vi "Retrieve Buffered Currents.vi"(0 "VISA resource name in":refnum<visa-resource-name>, 7 "Expected Points?":i32, 11 "error in":errorcluster) -> (4 "VISA resource name out":refnum<visa-resource-name>, 8 "Current Data":sgl[](array[numeric]), 15 "error out":errorcluster)   [LabVIEW 2010]
uses:
  <instrlib>/Keithley 2400/Keithley 24XX.lvlib
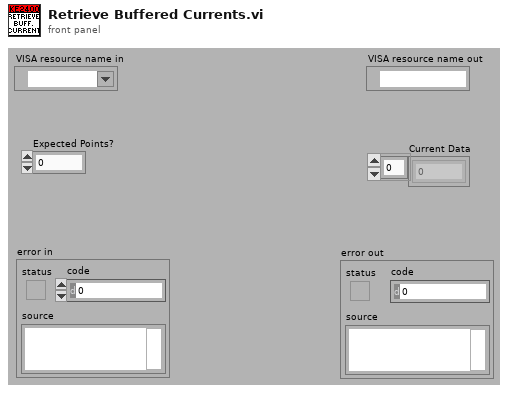
[diagram p1: front panel]
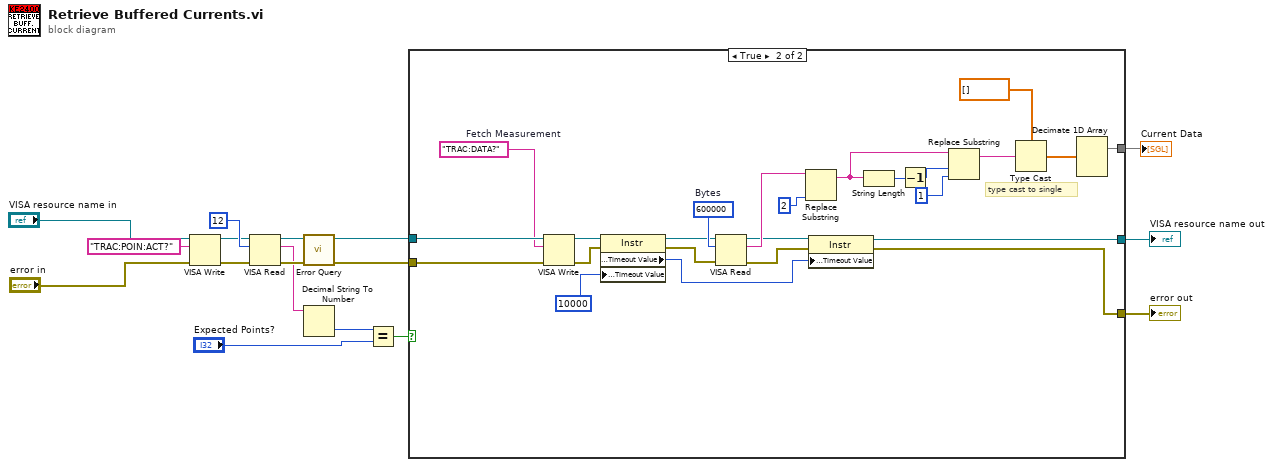
[diagram p0: block diagram]
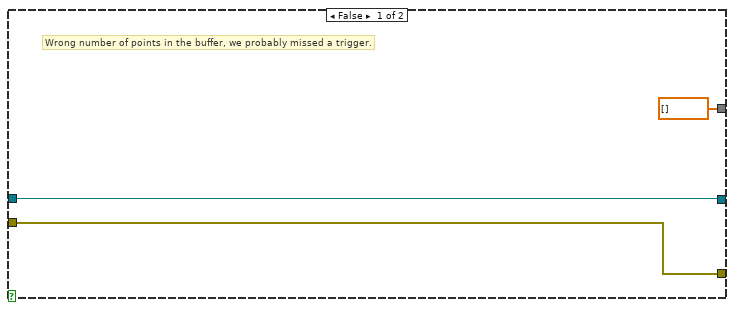
[diagram p2: hidden frame]
diagram:
  n1 = VISA Write(VISA resource name="VISA resource name in", write buffer="TRAC:POIN:ACT?", error in (no error)="error in") -> (VISA resource name out=w9:refnum<visa-resource-name>, error out=w8:errorcluster)  [unwired: 1 out]
  n2 = VISA Read(VISA resource name=w9, byte count=u32 12, error in (no error)=w8) -> (VISA resource name out=w10:refnum<visa-resource-name>, read buffer=w5:string, error out=w11:errorcluster)  [unwired: 1 out]
  n3 = call <instrlib>:"Error Query.vi"("error in (no error)"=w11, "VISA resource name"=w10) -> ("error out"=w16:errorcluster, "VISA resource name out"=w15:refnum<visa-resource-name>)  [unwired: 6 in, 2 out]
  n4 = Decimal String To Number(string=w5) -> (number=w4:i32)  [unwired: 2 in, 1 out]
  n5 = Equal?(x=w4, y="Expected Points?") -> (x = y?=w1:bool)
  n6 = case shown="True" w1 {
    tunnel: w16 -> [w19 w44]
    tunnel: w15 -> [w20 w43]
    tunnel: [w20 w41] -> w7
    tunnel: [w19 w40] -> w6
    tunnel: [sgl[] [] w21] -> w2
    frame False {
      # "Wrong number of points in the buffer, we probably missed a trigger."
    }
    frame True {
      w23 = "TRAC:DATA?"  # Fetch Measurement
      w30 = u32 600000  # Bytes
      # "type cast to single"
      n7 = VISA Write(VISA resource name=w43, write buffer=w23, error in (no error)=w44) -> (VISA resource name out=w31:refnum<visa-resource-name>, error out=w24:errorcluster)  [unwired: 1 out]
      n8 = property class="Instr"(reference=w31, error in=w24, "General Settings:Timeout Value"=u32 10000) -> (reference out=w25:refnum<visa-resource-name>, error out=w26:errorcluster, "General Settings:Timeout Value"=w29:u32)
      n9 = VISA Read(VISA resource name=w25, byte count=w30, error in (no error)=w26) -> (VISA resource name out=w27:refnum<visa-resource-name>, read buffer=w39:string, error out=w28:errorcluster)  [unwired: 1 out]
      n10 = Replace Substring(2:2 ("length (len. of substring)"), 5:w39) -> (1:w33:string)  [unwired: 2 in, 1 out]
      n11 = property class="Instr"(reference=w27, error in=w28, "General Settings:Timeout Value"=w29) -> (reference out=w41:refnum<visa-resource-name>, error out=w40:errorcluster)
      n12 = String Length(string=w33) -> (length=w34:i32)
      n13 = Decrement(x=w34) -> (x-1=w35:i32)
      n14 = Replace Substring(2:1 ("length (len. of substring)"), 3:w35, 5:w33) -> (1:w37:string)  [unwired: 1 in, 1 out]
      n15 = Type Cast(type=sgl[] [], x=w37) -> (*(type *) &x=w22:sgl[])
      n16 = Decimate 1D Array(w22) -> (w21:sgl[])  [unwired: 4 out]
    }
  }
  "VISA resource name out" <- w7
  "error out" <- w6
  "Current Data" <- w2
